vi "Speichern vorbereiten.vi"(7 "Neue Daten":string[](array[string]), 8 "Index":i16, 10 "LogFile Daten":string[][](array[string]), 11 "Speicherpfad":path) -> (0 "Index":i16, 2 "LogFile Daten":string[][](array[string]), 3 "Speicherpfad":path, 4 "error out":errorcluster)   [LabVIEW 2020, in "LogKonfig.lvlib"]
uses:
  LogKonfig.lvlib
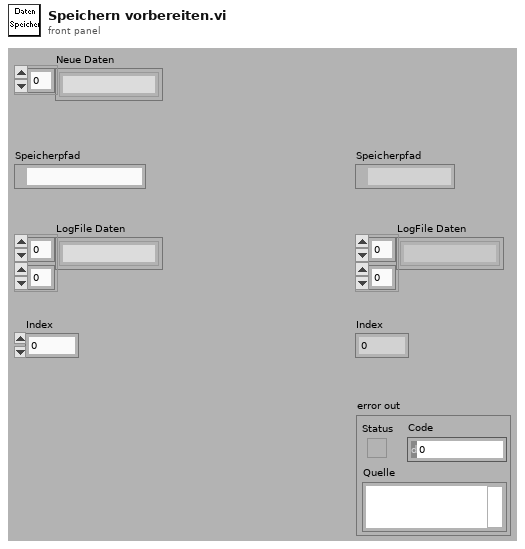
[diagram p1: front panel]
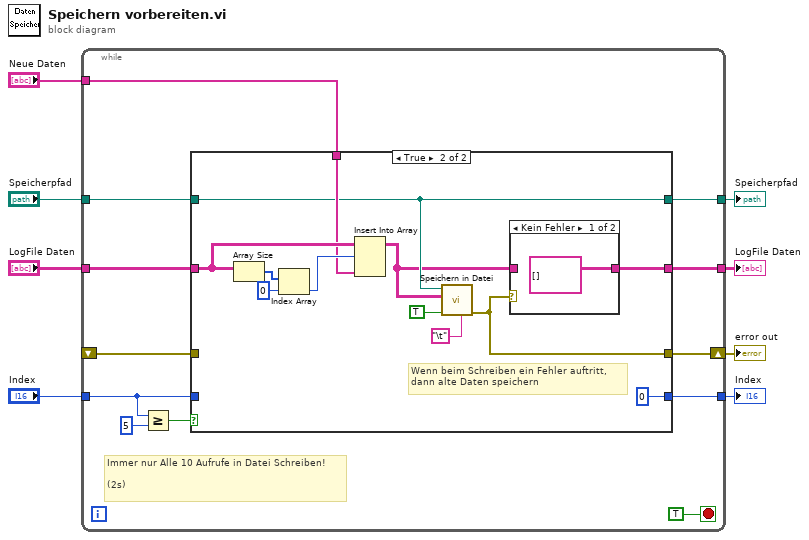
[diagram p0: block diagram]
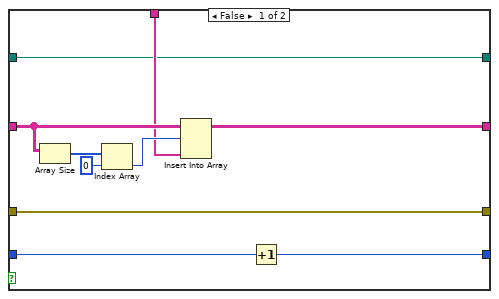
[diagram p2: hidden frame]
diagram:
  n1 = while {
    tunnel: "Index" -> [w19]
    tunnel: "LogFile Daten" -> [w17]
    tunnel: "Speicherpfad" -> [w16]
    tunnel: "Neue Daten" -> [w15]
    tunnel: [w14] -> w4
    tunnel: [w13] -> w3
    tunnel: [w12] -> w2
    shift-right: [w10] -> w1
    shift-left: _ -> [w9]
    stop <- TRUE stop-if-true
    # "Immer nur Alle 10 Aufrufe in Datei Schreiben!\n\n(2s)"
    n2 = Greater Or Equal?(x=w19, y=i16 5 ("Index")) -> (x >= y?=w18:bool)
    n3 = case shown="True" w18 {
      tunnel: w17 -> [w27 w39]
      tunnel: w15 -> [w25 w38]
      tunnel: [w26 w34] -> w13
      tunnel: w16 -> [w22 w36]
      tunnel: w19 -> [w24 _]
      tunnel: [w23 i16 0 ("Index")] -> w14
      tunnel: [w22 w36] -> w12
      tunnel: [w21 w32] -> w10
      tunnel: w9 -> [w21 _]
      frame False {
        n4 = Array Size(array=w27) -> (size(s)=w30:i32[])
        n5 = Index Array(array=w30, index=0 ("Index")) -> (element=w28:i32)
        n6 = Insert Into Array(array=w27, index (row)=w28, new element=w25) -> (w26:string[][])  [unwired: 1 in]
        n7 = Increment(x=w24) -> (x+1=w23:i16)
      }
      frame True {
        # "Wenn beim Schreiben ein Fehler auftritt, \ndann alte Daten speichern"
        n8 = Array Size(array=w39) -> (size(s)=w40:i32[])
        n9 = Index Array(array=w40, index=0 ("Index")) -> (element=w42:i32)
        n10 = Insert Into Array(array=w39, index (row)=w42, new element=w38) -> (w33:string[][])  [unwired: 1 in]
        n11 = call "Speichern in Datei.vi"("delimiter (\\t)"="\t", "append to file? (new file:F)"=TRUE, "2D data"=w33, "file path (dialog if empty)"=w36) -> ("error out"=w32:errorcluster)  [unwired: 6 in, 1 out]
        n12 = case shown="Kein Fehler" w32 {
          tunnel: [string[][] [] ("Angehängtes Array") w44] -> w34
          tunnel: w33 -> [_ w44]
          frame No Error {
          }
          frame Error {
          }
        }
      }
    }
  }
  "Speicherpfad" <- w2
  "LogFile Daten" <- w3
  "Index" <- w4
  "error out" <- w1
